vi "Write Proto Test Configuration.vi"(8 "error in (no error)":errorcluster, 10 "Cluster":T1, 11 "Protocol Verification Test in":refnum<class "Protocol Verification Test.lvclass">) -> (0 "error out":errorcluster, 3 "Protocol Verification Test out":refnum<class "Protocol Verification Test.lvclass">)   [LabVIEW 2017, in "Protocol Verification Test.lvlib" / "Protocol Verification Test.lvclass"]
uses:
  Protocol Verification Test.lvclass
  Protocol Verification Configuration.ctl
  Protocol Verification Test.lvclass/Protocol Verification Test.ctl
  Protocol Verification Test.lvlib
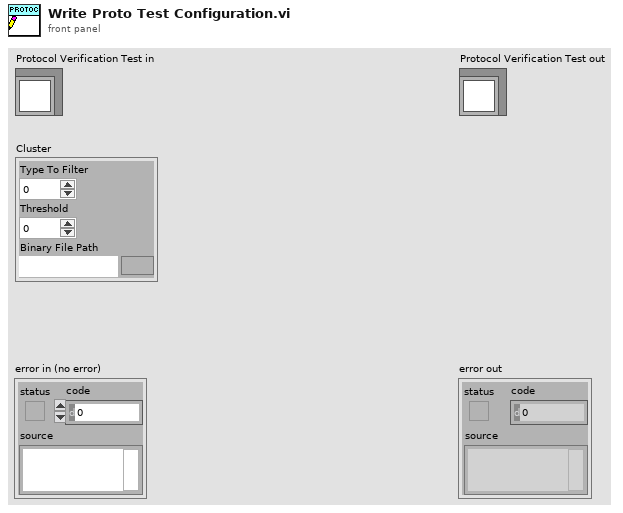
[diagram p1: front panel]
types:
  T1 = typedef "Protocol Verification Test.lvlib/Protocol Verification Configuration.ctl" = cluster{"Type To Filter":i32, "Threshold":dbl, "Binary File Path":path}
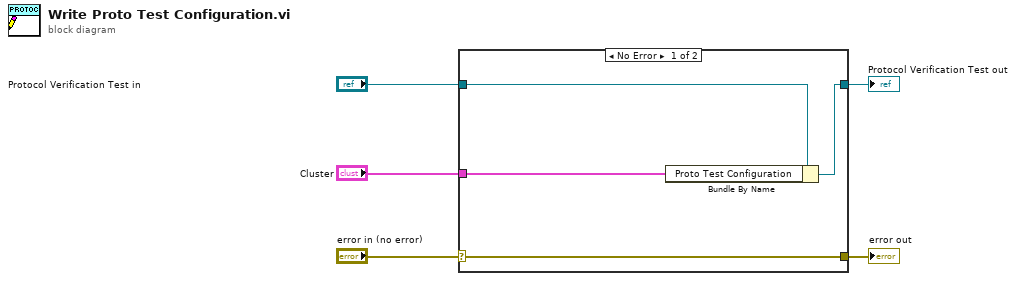
[diagram p0: block diagram]
diagram:
  n1 = case shown="No Error" "error in (no error)" {
    selector: "error in (no error)" -> [w9 w10]
    tunnel: [w9 w10] -> w4
    tunnel: [w7 w11] -> w2
    tunnel: "Protocol Verification Test in" -> [w8 w11]
    tunnel: "Cluster" -> [w6 _]
    frame No Error {
      n2 = Bundle By Name(cluster=w8, "Proto Test Configuration"=w6) -> (w7:refnum<class "Protocol Verification Test.lvclass">)
    }
    frame Error {
    }
  }
  "error out" <- w4
  "Protocol Verification Test out" <- w2
